vi "WriteServiceDetails.vi"(8 "error in (no error)":errorcluster, 10 "ServiceDetails":T1, 11 "MicronGRPCClient in":refnum<class "MicronGRPCClient.lvclass">) -> (0 "error out":errorcluster, 3 "MicronGRPCClient out":refnum<class "MicronGRPCClient.lvclass">)   [LabVIEW 2019, in "MicronGRPCClient.lvclass"]
uses:
  MicronGRPCClient.lvclass
  Base/Client/Typedefs/ServiceDetails.ctl
  MicronGRPCClient.lvclass/MicronGRPCClient.ctl
  Base/Client/MicronClient.lvclass
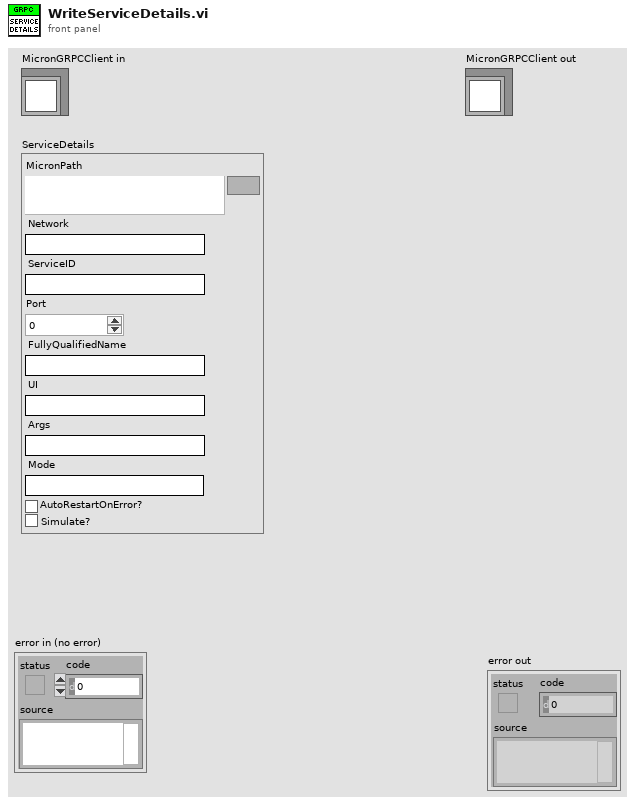
[diagram p1: front panel]
types:
  T1 = typedef "MicronClient.lvclass/ServiceDetails.ctl" = cluster{"MicronPath":path, "Network":string, "ServiceID":string, "Port":i32, "FullyQualifiedName":string, "UI":string, "Args":string, "Mode":string, "AutoRestartOnError?":bool, "Simulate?":bool}
  T2 = typedef "MicronGRPCClient.lvclass/InternalCluster.ctl" = cluster{"ServiceDetails":T1, "gRPCDetails":T3}
  T3 = typedef "gRPCDetails.ctl" = cluster{"ConnectionString":string, "ID":T4, "PackageName":string, "ServiceName":string}
  T4 = typedef "grpc-lvsupport-release.lvlib/grpcId.ctl" = u64
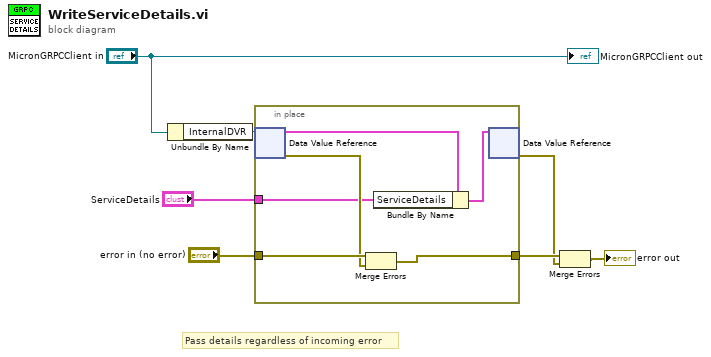
[diagram p0: block diagram]
diagram:
  # "Pass details regardless of incoming error"
  n1 = Unbundle By Name("MicronGRPCClient in") -> ("InternalDVR"=w7:refnum<data-value>)
  n2 = in-place {
    in-place-border: "error in (no error)" -> [w13]
    in-place-border: [w11] -> w6
    in-place-border: "ServiceDetails" -> [w8]
    n3 = in-place-dvr #1(w7) -> (w10:T2, w12:errorcluster)
    n4 = Merge Errors(w13, w12) -> (w11:errorcluster)
    n5 = Bundle By Name(cluster=w10, "ServiceDetails"=w8) -> (w9:T2)
    n6 = in-place-dvr #1(w9) -> (w5:errorcluster)  [unwired: 1 out]
  }
  n7 = Merge Errors(w6, w5) -> (→"error out":errorcluster)
  "MicronGRPCClient out" <- "MicronGRPCClient in"
